vi "Keypress.vi"() -> ()   [LabVIEW 2021]
panel:
  out "Key pressed":i16
  out "turn":dbl
  out "Vref":dbl
  out "Num_3_presses":dbl
  out "Num_r_presses":dbl
  out "Num_q_presses":dbl
  in  "stop":bool
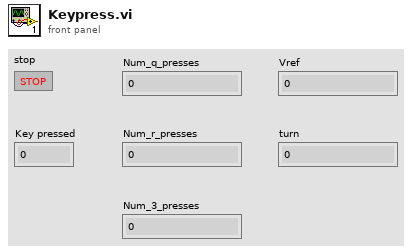
[diagram p1: front panel]
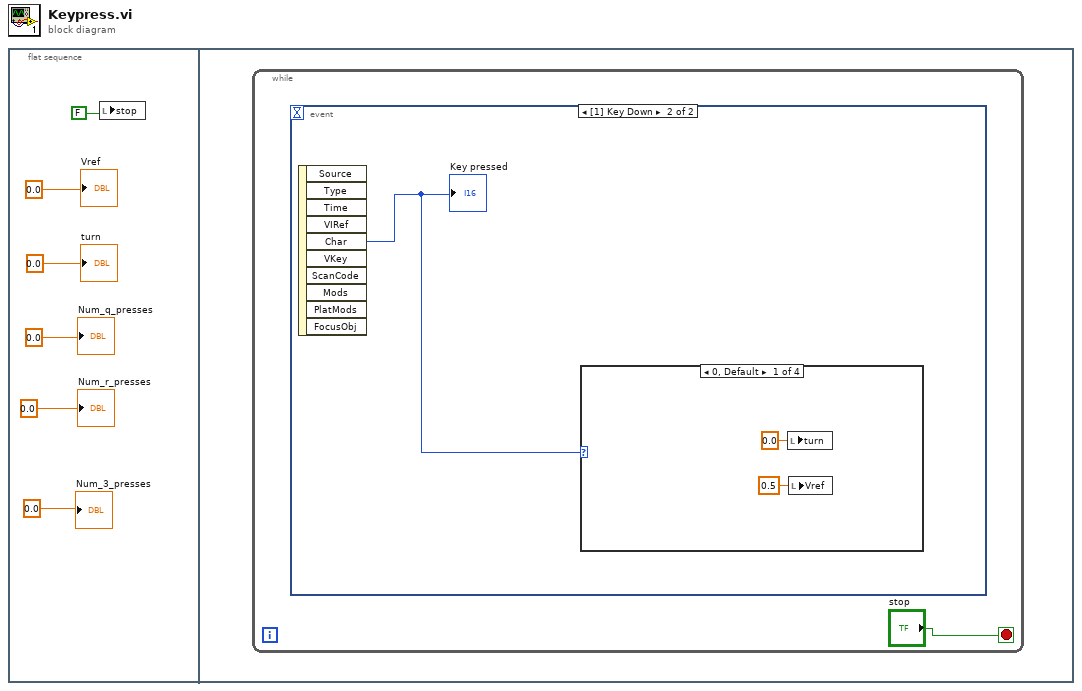
[diagram p0: block diagram]
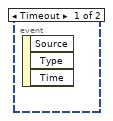
[diagram p2: hidden frame]
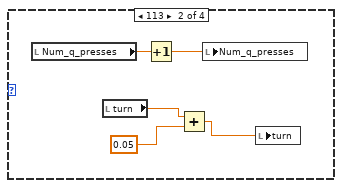
[diagram p3: hidden frame]
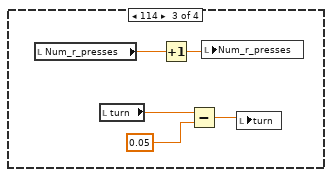
[diagram p4: hidden frame]
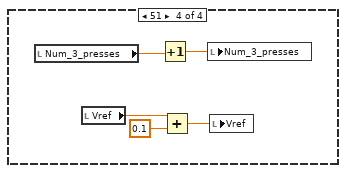
[diagram p5: hidden frame]
diagram:
  n1 = flat-sequence {
    frame #0 {
      n2 = local write "stop"(FALSE) -> ()
      "Num_q_presses" <- 0.0
      "Num_r_presses" <- 0.0
      "Num_3_presses" <- 0.0
      "Vref" <- 0.0
      "turn" <- 0.0
    }
    frame #1 {
      n3 = while {
        stop <- "stop" stop-if-true
        n4 = event shown="[1] Key Down" {
          selector: _ -> [_ _]
          dyn-events: _ -> [_ _]
          timeout: _ -> [_ _]
          event Timeout {
            n5 = event-data() -> ()  [unwired: 1 in, 3 out]
          }
          event Key Down {
            n6 = event-data() -> ("Char"=w8:i16)  [unwired: 1 in, 9 out]
            "Key pressed" <- w8
            n7 = case shown="0, Default" w8 {
              frame 0, Default {
                n8 = local write "turn"(0.0 ("turn")) -> ()
                n9 = local write "Vref"(0.5 ("Vref")) -> ()
              }
              frame 113 {
                n10 = local read "Num_q_presses"() -> (w15:dbl)
                n11 = local read "turn"() -> (w13:dbl)
                n12 = Increment(x=w15) -> (x+1=w14:dbl)
                n13 = Add(x=w13, y=0.05) -> (x+y=w12:dbl)
                n14 = local write "Num_q_presses"(w14) -> ()
                n15 = local write "turn"(w12) -> ()
              }
              frame 114 {
                n16 = local read "Num_r_presses"() -> (w16:dbl)
                n17 = local read "turn"() -> (w18:dbl)
                n18 = Increment(x=w16) -> (x+1=w20:dbl)
                n19 = Subtract(x=w18, y=0.05) -> (x-y=w19:dbl)
                n20 = local write "Num_r_presses"(w20) -> ()
                n21 = local write "turn"(w19) -> ()
              }
              frame 51 {
                n22 = local read "Num_3_presses"() -> (w21:dbl)
                n23 = local read "Vref"() -> (w24:dbl)
                n24 = Increment(x=w21) -> (x+1=w22:dbl)
                n25 = Add(x=w24, y=0.1) -> (x+y=w25:dbl)
                n26 = local write "Num_3_presses"(w22) -> ()
                n27 = local write "Vref"(w25) -> ()
              }
            }
          }
        }
      }
    }
  }
